vi "Write Auto-init.vi"(8 "error in (no error)":errorcluster, 10 "Auto-init":bool, 11 "Keithley Driver in":refnum<class "Keithley Driver.lvclass">) -> (0 "error out":errorcluster, 3 "Keithley Driver out":refnum<class "Keithley Driver.lvclass">)   [LabVIEW 2019, in "Keithley Driver.lvclass"]
uses:
  Keithley Driver.lvclass
  Keithley Driver.lvclass/Keithley Driver.ctl
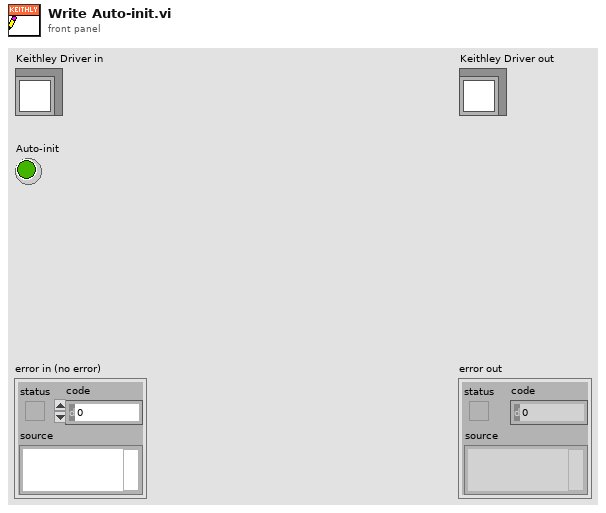
[diagram p1: front panel]
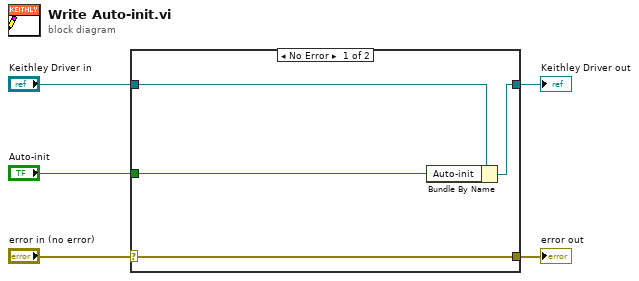
[diagram p0: block diagram]
diagram:
  n1 = case shown="No Error" "error in (no error)" {
    selector: "error in (no error)" -> [w9 w10]
    tunnel: [w9 w10] -> w4
    tunnel: [w7 w11] -> w2
    tunnel: "Keithley Driver in" -> [w8 w11]
    tunnel: "Auto-init" -> [w6 _]
    frame No Error {
      n2 = Bundle By Name(cluster=w8, "Auto-init"=w6) -> (w7:refnum<class "Keithley Driver.lvclass">)
    }
    frame Error {
    }
  }
  "error out" <- w4
  "Keithley Driver out" <- w2
